vi "Init Runtime.vi"(8 "error in (no error)":errorcluster, 10 "data allocations":T1, 11 "Wait Step Config in":refnum<class "Wait Step Config.lvclass">) -> (0 "error out":errorcluster, 2 "Skip":bool, 3 "Wait Step Config out":refnum<class "Wait Step Config.lvclass">)   [LabVIEW 2015, in "Wait Step Config.lvclass"]
uses:
  Wait Step Config.lvclass
  <vilib>/NI/Tag Bus Module Framework/channel/data tables.ctl
  <vilib>/NI/Tag Bus/dictionary/data dictionary.lvclass
  <vilib>/NI/Tag Bus/dictionary table pair.ctl
  <vilib>/NI/Tag Bus/table/data table.ctl
  Wait Step/Wait Step.lvclass
  <vilib>/NI/Tag Bus/table/data table.lvlib
  <vilib>/NI/Tag Bus/tag bus.lvlib
  <vilib>/NI/Tag Bus Module Framework/channel/TBM channel.lvclass
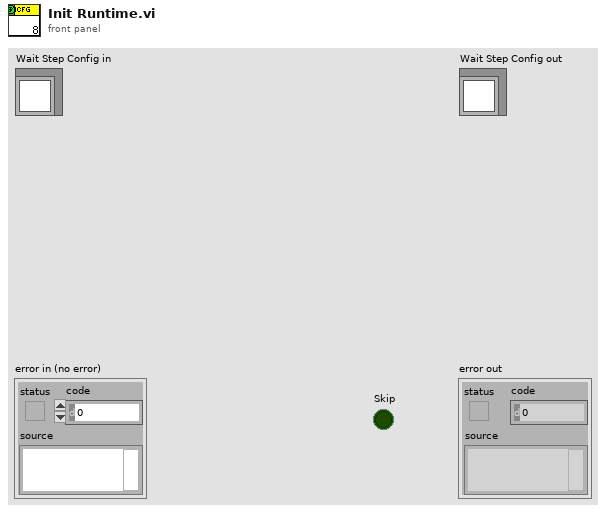
[diagram p1: front panel]
types:
  T1 = typedef "TBM channel.lvclass/data tables.ctl" = cluster{"input data":T2, "processing parameter":T2, "processing result":T2, "output data":T2}
  T2 = typedef "tag bus.lvlib/dictionary table pair.ctl" = cluster{"data dictionary":refnum<class "data dictionary.lvclass">, "data table":T3}
  T3 = typedef "tag bus.lvlib/data table.lvlib/data table.ctl" = cluster{"Double":dbl[], "Single":sgl[], "I64":i64[], "I32":i32[], "I16":i16[], "I8":i8[], "U64":u64[], "U32":u32[], "U16":u16[], "U8":u8[], "Boolean":bool[], "String":string[], "Array of Double":cluster{"DBL Array":dbl[]}[], "Array of Single":cluster{"SGL Array":sgl[]}[], "Array of I64":cluster{"I64 Array":i64[]}[], "Array of I32":cluster{"I32 Array":i32[]}[], "Array of I16":cluster{"I16 Array":i16[]}[], "Array of I8":cluster{"I8 Array":i8[]}[], "Array of U64":cluster{"U64 Array":u64[]}[], "Array of U32":cluster{"U32 Array":u32[]}[], "Array of U16":cluster{"U16 Array":u16[]}[], "Array of U8":cluster{"U8 Array":u8[]}[], "Array of Boolean":cluster{"Boolean Array":bool[]}[], "Array of String":cluster{"String Array":string[]}[]}
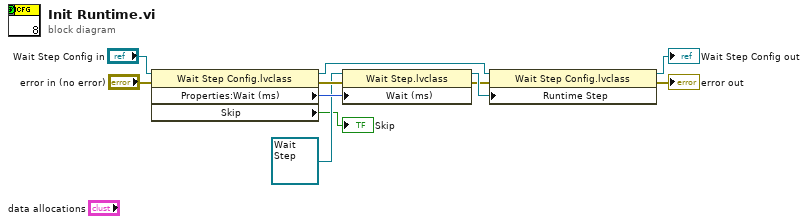
[diagram p0: block diagram]
diagram:
  n1 = property class="Wait Step Config.lvclass"(reference="Wait Step Config in", error in="error in (no error)") -> (reference out=w10:refnum<class "Wait Step Config.lvclass">, error out=w5:errorcluster, "Properties:Wait (ms)"=w7:u32, "Skip"=→"Skip":bool)
  n2 = property class="Wait Step.lvclass"(reference=refnum<class "Wait Step.lvclass"> refnum ("Wait Step.lvclass"), error in=w5, "Wait (ms)"=w7) -> (reference out=w8:refnum<class "Wait Step.lvclass">, error out=w4:errorcluster)
  n3 = property class="Wait Step Config.lvclass"(reference=w10, error in=w4, "Runtime Step"=w8) -> (reference out=→"Wait Step Config out":refnum<class "Wait Step Config.lvclass">, error out=→"error out":errorcluster)
